vi "Read N Swipe Directions.vi"(8 "Error In":errorcluster, 11 "Leap Handle":T3) -> (0 "Error Out":errorcluster, 1 "Swipe Statuses":T2[](array[typedef]), 2 "Swipe Directions":T1[](array[typedef]), 3 "Leap Handle":T3)   [LabVIEW 2011, in "LVH-Leap.lvlib"]
uses:
  LVH-Leap.lvlib
  Private/Type Defs/Leap Handle.ctl
  C:/github/labviewhacker/LVH-Leap/LabVIEW/vi.lib/LabVIEW Hacker/Leap/Private/Libs/LeapCSharp.NET3.5.dll
  Private/Libs/LeapCSharp.NET3.5.dll
  Private/Type Defs/Gesture State.ctl
  Private/Type Defs/Swipe Direction.ctl
  Read N Swipes.vi
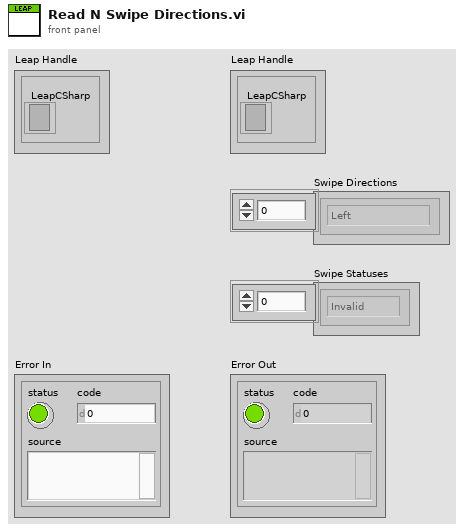
[diagram p1: front panel]
types:
  T1 = typedef "LVH-Leap.lvlib/Swipe Direction.ctl" = enum16{"Left", "Right", "Up", "Down", "In", "Out"}
  T2 = typedef "LVH-Leap.lvlib/Gesture State.ctl" = enum16{"Invalid", "Start", "Update", "Stop"}
  T3 = typedef "LVH-Leap.lvlib/Leap Handle.ctl" = cluster{"LeapCSharp":refnum<k24>}
  T4 = typedef "LVH-Leap.lvlib/Gesture Swipe.ctl" = cluster{"Common":T5, "Direction":T7, "Position":T7, "Start Position":T7, "Speed":dbl}
  T5 = typedef "LVH-Leap.lvlib/Gesture Common.ctl" = cluster{"ID":dbl, "Duration (S)":dbl, "Gesture Type":T6, "Gesture State":T2}
  T6 = typedef "LVH-Leap.lvlib/Gesture Type.ctl" = enum16{"Invalid", "Swipe", "Circle", "Screen Tap", "Key Tap"}
  T7 = typedef "LVH-Leap.lvlib/Vector.ctl" = cluster{"Pitch":sgl, "Yaw":sgl, "Roll":sgl, "Magnitude":sgl, "XYZ":sgl[]}
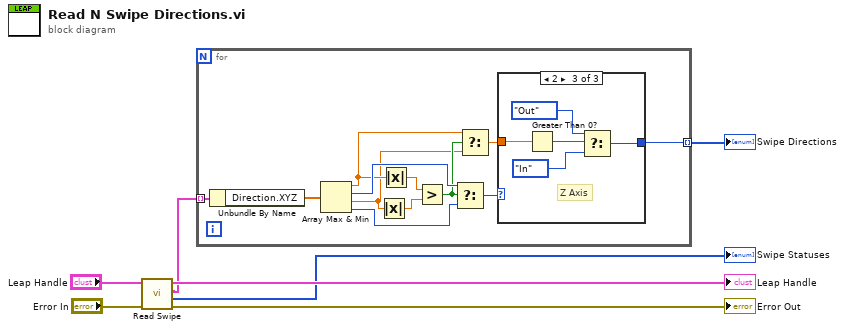
[diagram p0: block diagram]
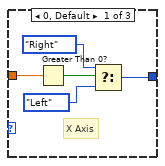
[diagram p2: hidden frame]
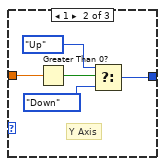
[diagram p3: hidden frame]
diagram:
  n1 = call-poly "Read Swipe.vi"("Error In"="Error In", "Leap Handle"="Leap Handle") -> ("Error Out"=→"Error Out":errorcluster, "Swipe Statuses"=→"Swipe Statuses":T2[], "Swipe Gestures"=w5:T4[], "Leap Handle"=→"Leap Handle":T3)  [unwired: 6 in]
  n2 = for {
    tunnel: w5 -> [w19] mode=indexing
    tunnel: [w8] -> w1 mode=indexing
    n3 = Unbundle By Name(w19) -> ("Direction.XYZ"=w18:sgl[])
    n4 = Array Max & Min(array=w18) -> (max value=w11:sgl, max index (indices)=w15:i32, min value=w10:sgl, min index (indices)=w14:i32)
    n5 = Absolute Value(x=w10) -> (abs(x)=w16:sgl)
    n6 = Absolute Value(x=w11) -> (abs(x)=w17:sgl)
    n7 = Greater?(x=w17, y=w16) -> (0:w12:bool)
    n8 = Select(t=w15, s=w12, f=w14) -> (s? t:f=w13:i32)
    n9 = Select(t=w11, s=w12, f=w10) -> (s? t:f=w9:sgl)
    n10 = case shown="2" w13 {
      tunnel: w9 -> [w24 w29 w34]
      tunnel: [w20 w25 w30] -> w8
      frame 0, Default {
        # "X Axis"
        n11 = Greater Than 0?(x=w24) -> (x > 0?=w23:bool)
        n12 = Select(t=Swipe_Direction."Right" ("Swipe Direction"), s=w23, f=Swipe_Direction."Left" ("Swipe Direction")) -> (s? t:f=w20:T1)
      }
      frame 1 {
        # "Y Axis"
        n13 = Greater Than 0?(x=w29) -> (x > 0?=w28:bool)
        n14 = Select(t=Swipe_Direction."Up" ("Swipe Direction"), s=w28, f=Swipe_Direction."Down" ("Swipe Direction")) -> (s? t:f=w25:T1)
      }
      frame 2 {
        # "Z Axis"
        n15 = Greater Than 0?(x=w34) -> (x > 0?=w33:bool)
        n16 = Select(t=Swipe_Direction."Out" ("Swipe Direction"), s=w33, f=Swipe_Direction."In" ("Swipe Direction")) -> (s? t:f=w30:T1)
      }
    }
  }
  "Swipe Directions" <- w1
